vi "Main.vi"(8 "error in (no error)":errorcluster) -> (0 "error out":errorcluster)   [LabVIEW 2018, in "JSON to LVConstant Test.lvlib"]
uses:
  JSON to LVConstant Test.lvlib
  <vilib>/addons/_JKI Toolkits/Caraya/classes/Test/Test.lvclass
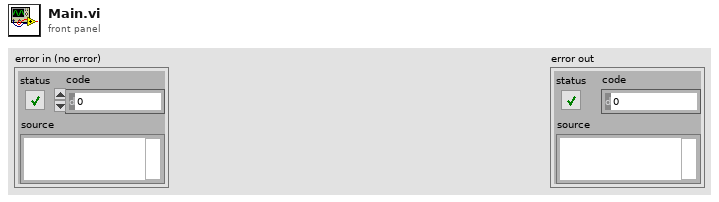
[diagram p1: front panel]
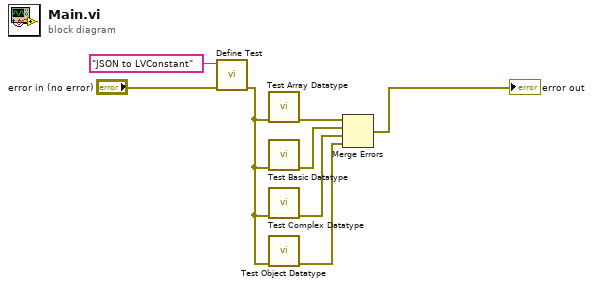
[diagram p0: block diagram]
diagram:
  n1 = call <vilib>:"Define Test.vi"("error in (no error)"="error in (no error)", "Label (VI Title)"="JSON to LVConstant") -> ("error out"=w8:errorcluster)  [unwired: 9 in]
  n2 = call "Test Array Datatype.vi"("error in (no error)"=w8) -> ("error out"=w6:errorcluster)  [unwired: 10 in]
  n3 = call "Test Basic Datatype.vi"("error in (no error)"=w8) -> ("error out"=w5:errorcluster)  [unwired: 10 in]
  n4 = call "Test Complex Datatype.vi"("error in (no error)"=w8) -> ("error out"=w4:errorcluster)  [unwired: 10 in]
  n5 = call "Test Object Datatype.vi"("error in (no error)"=w8) -> ("error out"=w3:errorcluster)  [unwired: 10 in]
  n6 = Merge Errors(w6, w5, w4, w3) -> (→"error out":errorcluster)
